vi "Manual Filenames.vi"(8 "Fehler (Eingang)":errorcluster, 9 "Flags Cluster":T4={"PDF Optionen (Eingang)"={"PDF Einzelseiten Komponenten"=FALSE, "PDF Einzelseiten Span"=FALSE, "PDF Deckblatt"=FALSE, "PDF öffnen"=FALSE, "Graphik für Messwerte"=FALSE}, "File Name LIN in"="", "Pfad LIN in"=path "", "active SPAN Idx out"=0, "Comp Idx out"=0, "1. Komponente"=TRUE, "Filename Overrride"=TRUE}, 10 "Zeitstempel":timestamp, 11 "SpanInletClusterArray in":T9[](array[typedef]) {"zusätzliche Zeitdauer Erster Punkt" min=30 step=1 format="%#_5g"; "Zeitdauer Stufen" format="%#_5g"; "Max Fehler" format="%#_5g"; "Anzahl Stufen" format="%#_5g"; "Komponenten"."Komponente 5"."Komponente:" items=["NO (350,3000) LP 191C", "NO2 (150) LP 191C (1of2)", "NO2 (2000) LP 191C (2of2)", "N2O (300) LP 191C (1of2)", "NH3 (300) LP 191C (1of2)", "NH3 (900,3000) LP 191C (2of2)", "HNCO (400) 191C", "H2O% (30) LP 191C", "Formaldehyde (70,500) LP 191C", "CO2 low% (4) LP 191C (2of2)", "CO2% (20) LP 191C (1of2)", "CO (700) LP 191C (1of3)", "CO% (1) LP 191C (2of3)", "Propylene (1000) LP 191C", "Aromatic HC C7 (500) LP 191C", "Ethylene (1000) LP 191C", "CH4 (250) LP 191C (1of2)", "CH4 (5000) LP 191C (2of2)", "Ethane (1000) LP 191C", "Acetylene (1000) LP 191C", "HNO2 (20) 191C", "MeOH (1000) 191C", "CO% (10) LP 191C (3of3)", "Formic Acid (100) 191C", "SO2 (500) LP 191C", "Acetaldehyde (1000) LP 191C", "COS (100) LP 191C", "1,3 butadiene (100) LP 191C", "Oil as Octane (200) LP 191C", "N2O (1000) LP 191C (2of2)", "Propane (200) LP 191C", "NO2 autorange (2000)", "CO autorange (100000)", "CH4 autorange (5000)", "NH3 autorange (3000)", "Temp. Gascell", "Pressure Gascell", "sBeam@2500"]; "Komponenten"."Komponente 5"."Konzentration IST" format="%#.4f"; "Komponenten"."Komponente 5"."Genauigkeit" format="%#.1f"; "Komponenten"."Komponente 4"."Komponente:" items=["NO (350,3000) LP 191C", "NO2 (150) LP 191C (1of2)", "NO2 (2000) LP 191C (2of2)", "N2O (300) LP 191C (1of2)", "NH3 (300) LP 191C (1of2)", "NH3 (900,3000) LP 191C (2of2)", "HNCO (400) 191C", "H2O% (30) LP 191C", "Formaldehyde (70,500) LP 191C", "CO2 low% (4) LP 191C (2of2)", "CO2% (20) LP 191C (1of2)", "CO (700) LP 191C (1of3)", "CO% (1) LP 191C (2of3)", "Propylene (1000) LP 191C", "Aromatic HC C7 (500) LP 191C", "Ethylene (1000) LP 191C", "CH4 (250) LP 191C (1of2)", "CH4 (5000) LP 191C (2of2)", "Ethane (1000) LP 191C", "Acetylene (1000) LP 191C", "HNO2 (20) 191C", "MeOH (1000) 191C", "CO% (10) LP 191C (3of3)", "Formic Acid (100) 191C", "SO2 (500) LP 191C", "Acetaldehyde (1000) LP 191C", "COS (100) LP 191C", "1,3 butadiene (100) LP 191C", "Oil as Octane (200) LP 191C", "N2O (1000) LP 191C (2of2)", "Propane (200) LP 191C", "NO2 autorange (2000)", "CO autorange (100000)", "CH4 autorange (5000)", "NH3 autorange (3000)", "Temp. Gascell", "Pressure Gascell", "sBeam@2500"]; "Komponenten"."Komponente 4"."Konzentration IST" format="%#.4f"; "Komponenten"."Komponente 4"."Genauigkeit" format="%#.1f"; "Komponenten"."Komponente 3"."Komponente:" items=["NO (350,3000) LP 191C", "NO2 (150) LP 191C (1of2)", "NO2 (2000) LP 191C (2of2)", "N2O (300) LP 191C (1of2)", "NH3 (300) LP 191C (1of2)", "NH3 (900,3000) LP 191C (2of2)", "HNCO (400) 191C", "H2O% (30) LP 191C", "Formaldehyde (70,500) LP 191C", "CO2 low% (4) LP 191C (2of2)", "CO2% (20) LP 191C (1of2)", "CO (700) LP 191C (1of3)", "CO% (1) LP 191C (2of3)", "Propylene (1000) LP 191C", "Aromatic HC C7 (500) LP 191C", "Ethylene (1000) LP 191C", "CH4 (250) LP 191C (1of2)", "CH4 (5000) LP 191C (2of2)", "Ethane (1000) LP 191C", "Acetylene (1000) LP 191C", "HNO2 (20) 191C", "MeOH (1000) 191C", "CO% (10) LP 191C (3of3)", "Formic Acid (100) 191C", "SO2 (500) LP 191C", "Acetaldehyde (1000) LP 191C", "COS (100) LP 191C", "1,3 butadiene (100) LP 191C", "Oil as Octane (200) LP 191C", "N2O (1000) LP 191C (2of2)", "Propane (200) LP 191C", "NO2 autorange (2000)", "CO autorange (100000)", "CH4 autorange (5000)", "NH3 autorange (3000)", "Temp. Gascell", "Pressure Gascell", "sBeam@2500"]; "Komponenten"."Komponente 3"."Konzentration IST" format="%#.4f"; "Komponenten"."Komponente 3"."Genauigkeit" format="%#.1f"; "Komponenten"."Komponente 2"."Komponente:" items=["NO (350,3000) LP 191C", "NO2 (150) LP 191C (1of2)", "NO2 (2000) LP 191C (2of2)", "N2O (300) LP 191C (1of2)", "NH3 (300) LP 191C (1of2)", "NH3 (900,3000) LP 191C (2of2)", "HNCO (400) 191C", "H2O% (30) LP 191C", "Formaldehyde (70,500) LP 191C", "CO2 low% (4) LP 191C (2of2)", "CO2% (20) LP 191C (1of2)", "CO (700) LP 191C (1of3)", "CO% (1) LP 191C (2of3)", "Propylene (1000) LP 191C", "Aromatic HC C7 (500) LP 191C", "Ethylene (1000) LP 191C", "CH4 (250) LP 191C (1of2)", "CH4 (5000) LP 191C (2of2)", "Ethane (1000) LP 191C", "Acetylene (1000) LP 191C", "HNO2 (20) 191C", "MeOH (1000) 191C", "CO% (10) LP 191C (3of3)", "Formic Acid (100) 191C", "SO2 (500) LP 191C", "Acetaldehyde (1000) LP 191C", "COS (100) LP 191C", "1,3 butadiene (100) LP 191C", "Oil as Octane (200) LP 191C", "N2O (1000) LP 191C (2of2)", "Propane (200) LP 191C", "NO2 autorange (2000)", "CO autorange (100000)", "CH4 autorange (5000)", "NH3 autorange (3000)", "Temp. Gascell", "Pressure Gascell", "sBeam@2500"]; "Komponenten"."Komponente 2"."Konzentration IST" format="%#.4f"; "Komponenten"."Komponente 2"."Genauigkeit" format="%#.1f"; "Komponenten"."Komponente 1"."Komponente:" items=["NO (350,3000) LP 191C", "NO2 (150) LP 191C (1of2)", "NO2 (2000) LP 191C (2of2)", "N2O (300) LP 191C (1of2)", "NH3 (300) LP 191C (1of2)", "NH3 (900,3000) LP 191C (2of2)", "HNCO (400) 191C", "H2O% (30) LP 191C", "Formaldehyde (70,500) LP 191C", "CO2 low% (4) LP 191C (2of2)", "CO2% (20) LP 191C (1of2)", "CO (700) LP 191C (1of3)", "CO% (1) LP 191C (2of3)", "Propylene (1000) LP 191C", "Aromatic HC C7 (500) LP 191C", "Ethylene (1000) LP 191C", "CH4 (250) LP 191C (1of2)", "CH4 (5000) LP 191C (2of2)", "Ethane (1000) LP 191C", "Acetylene (1000) LP 191C", "HNO2 (20) 191C", "MeOH (1000) 191C", "CO% (10) LP 191C (3of3)", "Formic Acid (100) 191C", "SO2 (500) LP 191C", "Acetaldehyde (1000) LP 191C", "COS (100) LP 191C", "1,3 butadiene (100) LP 191C", "Oil as Octane (200) LP 191C", "N2O (1000) LP 191C (2of2)", "Propane (200) LP 191C", "NO2 autorange (2000)", "CO autorange (100000)", "CH4 autorange (5000)", "NH3 autorange (3000)", "Temp. Gascell", "Pressure Gascell", "sBeam@2500"]; "Komponenten"."Komponente 1"."Konzentration IST" format="%#.4f"; "Komponenten"."Komponente 1"."Genauigkeit" format="%#.1f"; "Ablaufdatum" format="%<%d.%m.%Y>T"; "Gasflasche" items=["----"=10000, "IAG NH3 3000"=0, "IAG NH3 200"=1, "IAG NH3 2000"=2, "IAG MG"=3, "IAG O2"=4]}) -> (0 "Fehler (Ausgang)":errorcluster, 1 "LogInfo-Cluster":T6 {"Gasflasche" items=["----"=10000, "IAG NH3 3000"=0, "IAG NH3 200"=1, "IAG NH3 2000"=2, "IAG MG"=3, "IAG O2"=4]}, 2 "Pfad LIN Cluster":cluster{"Pfad LIN SPAN":T1, "Pfad LIN":path}, 3 "SpanInletClusterArray out":T9[](array[typedef]) {"zusätzliche Zeitdauer Erster Punkt" min=30 step=1 format="%#_5g"; "Zeitdauer Stufen" format="%#_5g"; "Max Fehler" format="%#_5g"; "Anzahl Stufen" format="%#_5g"; "Komponenten"."Komponente 5"."Komponente:" items=["NO (350,3000) LP 191C", "NO2 (150) LP 191C (1of2)", "NO2 (2000) LP 191C (2of2)", "N2O (300) LP 191C (1of2)", "NH3 (300) LP 191C (1of2)", "NH3 (900,3000) LP 191C (2of2)", "HNCO (400) 191C", "H2O% (30) LP 191C", "Formaldehyde (70,500) LP 191C", "CO2 low% (4) LP 191C (2of2)", "CO2% (20) LP 191C (1of2)", "CO (700) LP 191C (1of3)", "CO% (1) LP 191C (2of3)", "Propylene (1000) LP 191C", "Aromatic HC C7 (500) LP 191C", "Ethylene (1000) LP 191C", "CH4 (250) LP 191C (1of2)", "CH4 (5000) LP 191C (2of2)", "Ethane (1000) LP 191C", "Acetylene (1000) LP 191C", "HNO2 (20) 191C", "MeOH (1000) 191C", "CO% (10) LP 191C (3of3)", "Formic Acid (100) 191C", "SO2 (500) LP 191C", "Acetaldehyde (1000) LP 191C", "COS (100) LP 191C", "1,3 butadiene (100) LP 191C", "Oil as Octane (200) LP 191C", "N2O (1000) LP 191C (2of2)", "Propane (200) LP 191C", "NO2 autorange (2000)", "CO autorange (100000)", "CH4 autorange (5000)", "NH3 autorange (3000)", "Temp. Gascell", "Pressure Gascell", "sBeam@2500"]; "Komponenten"."Komponente 5"."Konzentration IST" format="%#.4f"; "Komponenten"."Komponente 5"."Genauigkeit" format="%#.1f"; "Komponenten"."Komponente 4"."Komponente:" items=["NO (350,3000) LP 191C", "NO2 (150) LP 191C (1of2)", "NO2 (2000) LP 191C (2of2)", "N2O (300) LP 191C (1of2)", "NH3 (300) LP 191C (1of2)", "NH3 (900,3000) LP 191C (2of2)", "HNCO (400) 191C", "H2O% (30) LP 191C", "Formaldehyde (70,500) LP 191C", "CO2 low% (4) LP 191C (2of2)", "CO2% (20) LP 191C (1of2)", "CO (700) LP 191C (1of3)", "CO% (1) LP 191C (2of3)", "Propylene (1000) LP 191C", "Aromatic HC C7 (500) LP 191C", "Ethylene (1000) LP 191C", "CH4 (250) LP 191C (1of2)", "CH4 (5000) LP 191C (2of2)", "Ethane (1000) LP 191C", "Acetylene (1000) LP 191C", "HNO2 (20) 191C", "MeOH (1000) 191C", "CO% (10) LP 191C (3of3)", "Formic Acid (100) 191C", "SO2 (500) LP 191C", "Acetaldehyde (1000) LP 191C", "COS (100) LP 191C", "1,3 butadiene (100) LP 191C", "Oil as Octane (200) LP 191C", "N2O (1000) LP 191C (2of2)", "Propane (200) LP 191C", "NO2 autorange (2000)", "CO autorange (100000)", "CH4 autorange (5000)", "NH3 autorange (3000)", "Temp. Gascell", "Pressure Gascell", "sBeam@2500"]; "Komponenten"."Komponente 4"."Konzentration IST" format="%#.4f"; "Komponenten"."Komponente 4"."Genauigkeit" format="%#.1f"; "Komponenten"."Komponente 3"."Komponente:" items=["NO (350,3000) LP 191C", "NO2 (150) LP 191C (1of2)", "NO2 (2000) LP 191C (2of2)", "N2O (300) LP 191C (1of2)", "NH3 (300) LP 191C (1of2)", "NH3 (900,3000) LP 191C (2of2)", "HNCO (400) 191C", "H2O% (30) LP 191C", "Formaldehyde (70,500) LP 191C", "CO2 low% (4) LP 191C (2of2)", "CO2% (20) LP 191C (1of2)", "CO (700) LP 191C (1of3)", "CO% (1) LP 191C (2of3)", "Propylene (1000) LP 191C", "Aromatic HC C7 (500) LP 191C", "Ethylene (1000) LP 191C", "CH4 (250) LP 191C (1of2)", "CH4 (5000) LP 191C (2of2)", "Ethane (1000) LP 191C", "Acetylene (1000) LP 191C", "HNO2 (20) 191C", "MeOH (1000) 191C", "CO% (10) LP 191C (3of3)", "Formic Acid (100) 191C", "SO2 (500) LP 191C", "Acetaldehyde (1000) LP 191C", "COS (100) LP 191C", "1,3 butadiene (100) LP 191C", "Oil as Octane (200) LP 191C", "N2O (1000) LP 191C (2of2)", "Propane (200) LP 191C", "NO2 autorange (2000)", "CO autorange (100000)", "CH4 autorange (5000)", "NH3 autorange (3000)", "Temp. Gascell", "Pressure Gascell", "sBeam@2500"]; "Komponenten"."Komponente 3"."Konzentration IST" format="%#.4f"; "Komponenten"."Komponente 3"."Genauigkeit" format="%#.1f"; "Komponenten"."Komponente 2"."Komponente:" items=["NO (350,3000) LP 191C", "NO2 (150) LP 191C (1of2)", "NO2 (2000) LP 191C (2of2)", "N2O (300) LP 191C (1of2)", "NH3 (300) LP 191C (1of2)", "NH3 (900,3000) LP 191C (2of2)", "HNCO (400) 191C", "H2O% (30) LP 191C", "Formaldehyde (70,500) LP 191C", "CO2 low% (4) LP 191C (2of2)", "CO2% (20) LP 191C (1of2)", "CO (700) LP 191C (1of3)", "CO% (1) LP 191C (2of3)", "Propylene (1000) LP 191C", "Aromatic HC C7 (500) LP 191C", "Ethylene (1000) LP 191C", "CH4 (250) LP 191C (1of2)", "CH4 (5000) LP 191C (2of2)", "Ethane (1000) LP 191C", "Acetylene (1000) LP 191C", "HNO2 (20) 191C", "MeOH (1000) 191C", "CO% (10) LP 191C (3of3)", "Formic Acid (100) 191C", "SO2 (500) LP 191C", "Acetaldehyde (1000) LP 191C", "COS (100) LP 191C", "1,3 butadiene (100) LP 191C", "Oil as Octane (200) LP 191C", "N2O (1000) LP 191C (2of2)", "Propane (200) LP 191C", "NO2 autorange (2000)", "CO autorange (100000)", "CH4 autorange (5000)", "NH3 autorange (3000)", "Temp. Gascell", "Pressure Gascell", "sBeam@2500"]; "Komponenten"."Komponente 2"."Konzentration IST" format="%#.4f"; "Komponenten"."Komponente 2"."Genauigkeit" format="%#.1f"; "Komponenten"."Komponente 1"."Komponente:" items=["NO (350,3000) LP 191C", "NO2 (150) LP 191C (1of2)", "NO2 (2000) LP 191C (2of2)", "N2O (300) LP 191C (1of2)", "NH3 (300) LP 191C (1of2)", "NH3 (900,3000) LP 191C (2of2)", "HNCO (400) 191C", "H2O% (30) LP 191C", "Formaldehyde (70,500) LP 191C", "CO2 low% (4) LP 191C (2of2)", "CO2% (20) LP 191C (1of2)", "CO (700) LP 191C (1of3)", "CO% (1) LP 191C (2of3)", "Propylene (1000) LP 191C", "Aromatic HC C7 (500) LP 191C", "Ethylene (1000) LP 191C", "CH4 (250) LP 191C (1of2)", "CH4 (5000) LP 191C (2of2)", "Ethane (1000) LP 191C", "Acetylene (1000) LP 191C", "HNO2 (20) 191C", "MeOH (1000) 191C", "CO% (10) LP 191C (3of3)", "Formic Acid (100) 191C", "SO2 (500) LP 191C", "Acetaldehyde (1000) LP 191C", "COS (100) LP 191C", "1,3 butadiene (100) LP 191C", "Oil as Octane (200) LP 191C", "N2O (1000) LP 191C (2of2)", "Propane (200) LP 191C", "NO2 autorange (2000)", "CO autorange (100000)", "CH4 autorange (5000)", "NH3 autorange (3000)", "Temp. Gascell", "Pressure Gascell", "sBeam@2500"]; "Komponenten"."Komponente 1"."Konzentration IST" format="%#.4f"; "Komponenten"."Komponente 1"."Genauigkeit" format="%#.1f"; "Ablaufdatum" format="%<%d.%m.%Y>T"; "Gasflasche" items=["----"=10000, "IAG NH3 3000"=0, "IAG NH3 200"=1, "IAG NH3 2000"=2, "IAG MG"=3, "IAG O2"=4]}, 4 "File Name LIN":T3, 5 "Span_Name":string, 6 "File Name EPA":T3 caption="File Name", 7 "File Names":T5)   [LabVIEW 2020, in "Linearisierung v2.lvlib" / "SpanEinstellungen.lvlib"]
uses:
  SpanEinstellungen.lvlib
  Visualisierungs Elemente/String - Eingabefeld.ctl
  SpanInletCluster.ctl
  Seiten/System Einstellungen V2/Konfig Gasflasche.ctl
  Seiten/System Einstellungen V2/Analysatoren.ctl
  Seiten/System Einstellungen V2/Gasflasche Auswahl.ctl
  Komponentencluster mit Formel.ctl
  Komponentenauswahl mit Formel.ctl
  Einheit.ctl
  Seiten/System Einstellungen V2/Traegergas.ctl
  ErrorLogInfoCluster.ctl
  Visualisierungs Elemente/String - Ausgabefeld.ctl
  PDF Optionen.ctl
  Visualisierungs Elemente/Pfad-Eingabefeld.ctl
  <vilib>/regexp/Match Regular Expression.xnode
  Allgemein/allgemeine Sub-VIs.lvlib
  Seiten/System Einstellungen V2/System Einstellungen V2.lvlib
panel:
  out "Deckblatt LIN":string
  out "Deckblatt EPA":string
  # "sec"
  # "%"
  # "sec"
  # "Komponente"
  # "Formel"
  # "Konzentration"
  # "Einheit"
  # "Genauigkeit [%]"
  # "sec"
  # "%"
  # "sec"
  # "Komponente"
  # "Formel"
  # "Konzentration"
  # "Einheit"
  # "Genauigkeit [%]"
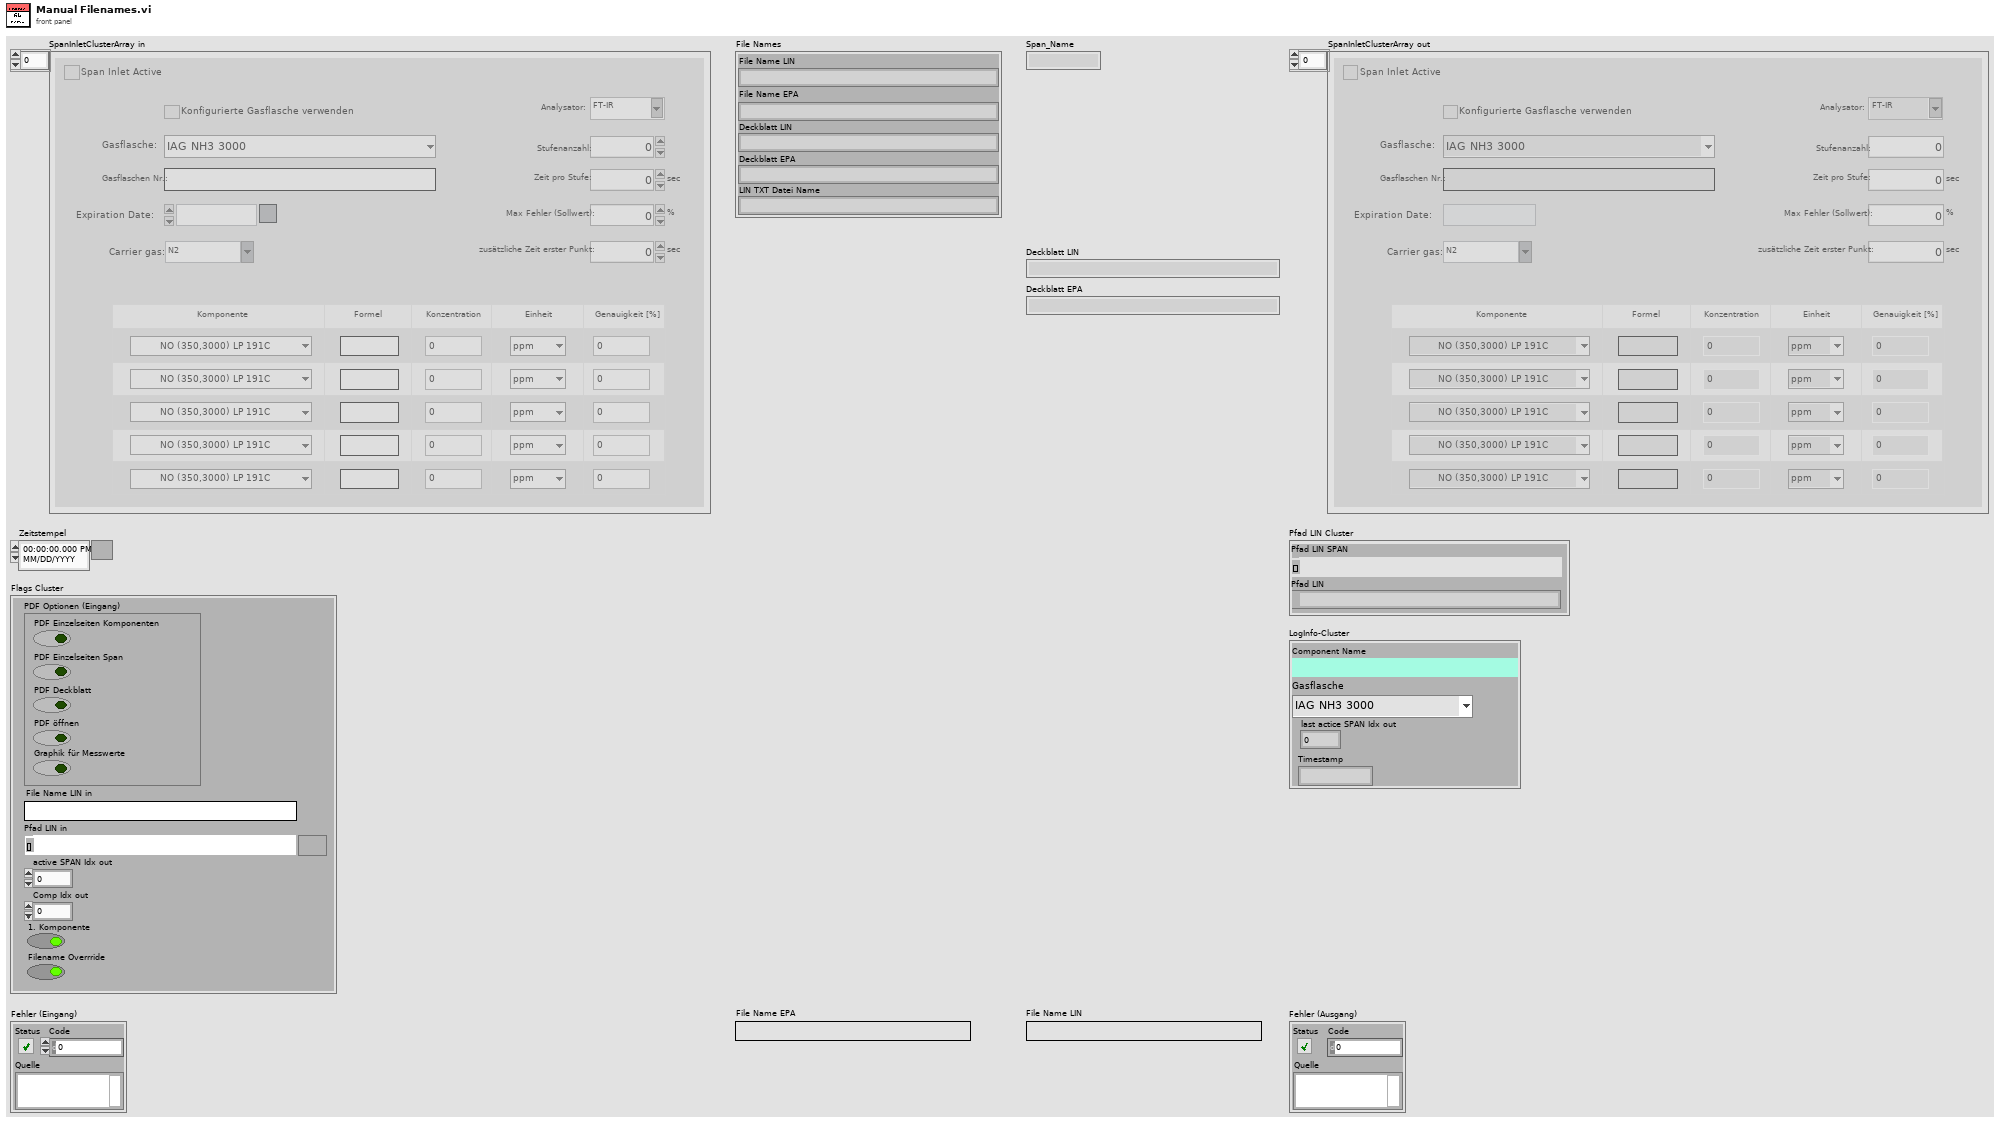
[diagram p1: front panel]
types:
  T1 = typedef "Pfad-Eingabefeld.ctl" = path
  T2 = typedef "Linearisierung v2.lvlib/SpanEinstellungen.lvlib/PDF Optionen.ctl" = cluster{"PDF Einzelseiten Komponenten":bool, "PDF Einzelseiten Span":bool, "PDF Deckblatt":bool, "PDF öffnen":bool, "Graphik für Messwerte":bool}
  T3 = typedef "String - Eingabefeld.ctl" = string
  T4 = cluster{"PDF Optionen (Eingang)":T2, "File Name LIN in":T3, "Pfad LIN in":T1, "active SPAN Idx out":i32, "Comp Idx out":i32, "1. Komponente":bool, "Filename Overrride":bool}
  T5 = cluster{"File Name LIN":string, "File Name EPA":string, "Deckblatt LIN":string, "Deckblatt EPA":string, "LIN TXT Datei Name":string}
  T6 = typedef "Linearisierung v2.lvlib/SpanEinstellungen.lvlib/ErrorLogInfoCluster.ctl" = cluster{"Component Name":T7, "Gasflasche":T8, "last actice SPAN Idx out":i32, "Timestamp":string}
  T7 = typedef "String - Ausgabefeld.ctl" = string
  T8 = typedef "System Einstellungen V2.lvlib/Gasflasche Auswahl.ctl" = u16
  T9 = typedef "Linearisierung v2.lvlib/SpanEinstellungen.lvlib/SpanInletCluster.ctl" = cluster{"Span Inlet Active":T10, "Analysator":T11, "Konfig Gasflasche":T10, "Gasflasche":T8, "Gasflaschen Nr.:":string, "Ablaufdatum":timestamp, "Komponenten":T12, "Zeitdauer Stufen":sgl, "Max Fehler":sgl, "Anzahl Stufen":sgl, "Trägergas":T15, "zusätzliche Zeitdauer Erster Punkt":sgl}
  T10 = typedef "System Einstellungen V2.lvlib/Konfig Gasflasche.ctl" = bool
  T11 = typedef "System Einstellungen V2.lvlib/Analysatoren.ctl" = string
  T12 = typedef "Linearisierung v2.lvlib/SpanEinstellungen.lvlib/Komponentencluster mit Formel.ctl" = cluster{"Komponente 1":T13, "Komponente 2":T13, "Komponente 3":T13, "Komponente 4":T13, "Komponente 5":T13}
  T13 = typedef "Linearisierung v2.lvlib/SpanEinstellungen.lvlib/Komponentenauswahl mit Formel.ctl" = cluster{"Komponente:":u16, "Summenformel":T3, "Konzentration IST":dbl, "Einheit":T14, "Genauigkeit":dbl}
  T14 = typedef "Linearisierung v2.lvlib/SpanEinstellungen.lvlib/Einheit.ctl" = enum16{"ppm", "%"}
  T15 = typedef "System Einstellungen V2.lvlib/Traegergas.ctl" = string
  T16 = cluster{"Component Name":T7, "Compnent Nr":u16, "Formelname(n)":string}
  T17 = cluster{"File Name LIN":string, "File Name EPA":string, "MG":bool}
  T18 = cluster{"Component Name":T7, "Gasflasche":T8, "active SPAN Idx out":i32, "date/time string":string}
  T19 = cluster{"File Name LIN in":T3, "File Name LIN in":T3, string, string, "File Name LIN":string}
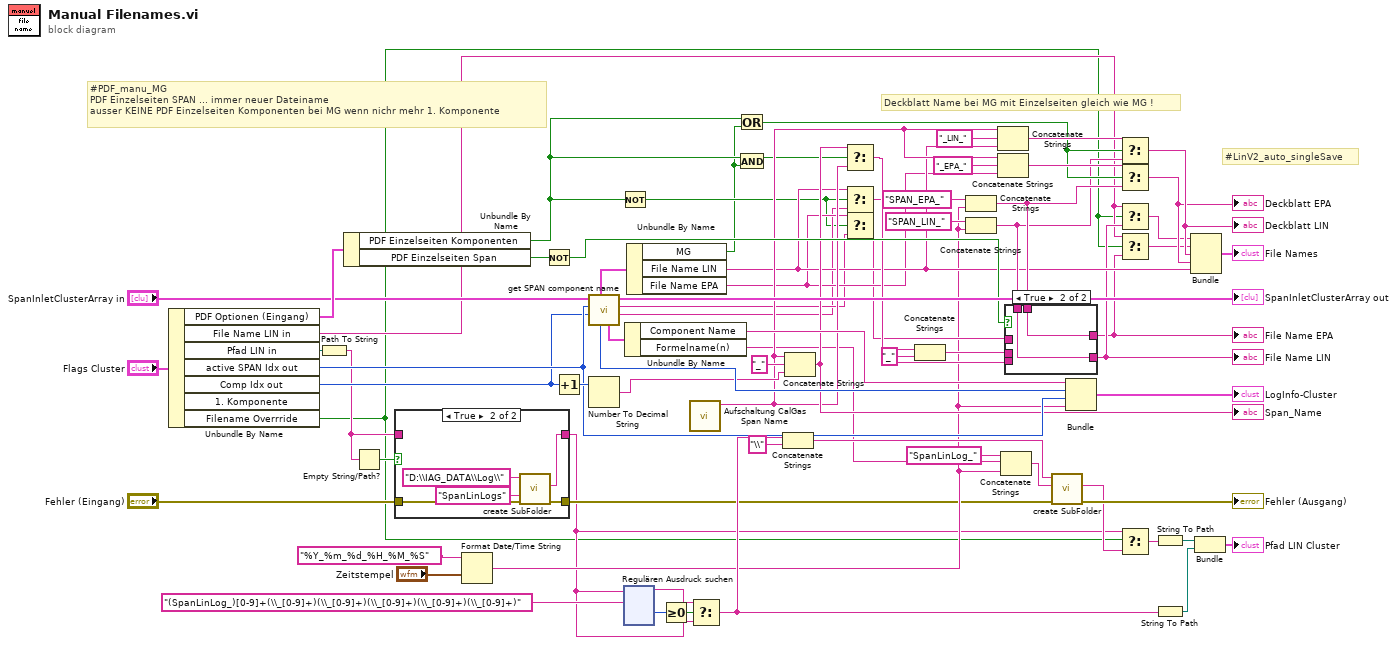
[diagram p0: block diagram]
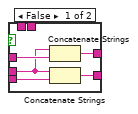
[diagram p3: hidden frame]
diagram:
  # "#LinV2_auto_singleSave"
  # "Deckblatt Name bei MG mit Einzelseiten gleich wie MG !"
  # "#PDF_manu_MG\nPDF Einzelseiten SPAN ... immer neuer Dateiname\nausser KEINE PDF Einzelseiten Komponenten bei MG wenn nichr mehr 1. Komponente"
  n1 = Unbundle By Name("Flags Cluster") -> ("PDF Optionen (Eingang)"=w60:T2, "File Name LIN in"=w5:T3, "Pfad LIN in"=w55:T1, "active SPAN Idx out"=w57:i32, "Comp Idx out"=w56:i32, "Filename Overrride"=w1:bool)  [unwired: 1 out]
  n2 = Path To String(path=w55) -> (string=w14:string)
  n3 = Unbundle By Name(w60) -> ("PDF Einzelseiten Komponenten"=w12:bool, "PDF Einzelseiten Span"=w53:bool)
  n4 = Empty String/Path?(string/path=w14) -> (empty?=w13:bool)
  n5 = case shown="True" w13 {
    tunnel: [w74 w80] -> w15
    tunnel: "Fehler (Eingang)" -> [w74 w79]
    tunnel: w14 -> [w75 _]
    tunnel: [w75 w76] -> w3
    frame False {
    }
    frame True {
      n6 = call "create SubFolder.vi"("Fehler (Eingang)"=w79, "Ordner"="SpanLinLogs", "Pfad"="D:\\IAG_DATA\\Log\\") -> ("Fehler (Ausgang)"=w80:errorcluster, "SubOrdner"=w76:string)  [unwired: 6 in, 1 out]
    }
  }
  n7 = Format Date/Time String(time format string (%c)="%Y_%m_%d_%H_%M_%S" ("Zeitformatierungs-String (%c)"), seconds (now)="Zeitstempel") -> (date/time string=w18:string)  [unwired: 1 in]
  n8 = Not(x=w53) -> (.not. x?=w50:bool)
  n9 = Increment(x=w56) -> (x+1=w65:i32)
  n10 = call "get SPAN component name.vi"("Comp Idx"=w56, "SPAN Idx"=w57, "SpanInletClusterArray in"="SpanInletClusterArray in") -> ("Protokoll Name LIN"=w30:string, "Protokoll Name EPA"=w31:string, "Komponente Nr Name -Cluster"=w69:T16, "Gasflasche"=w68:T8, "LIN/EPA TXT Datei Name"=w54:T17)  [unwired: 1 in, 3 out]
  n11 = Number To Decimal String(number=w65) -> (decimal integer string=w47:string)  [unwired: 1 in]
  n12 = Not(x=w12) -> (.not. x?=w27:bool)
  n13 = xnode "Regulären Ausdruck suchen"("Eingangs-String"=w3, "Regulärer Ausdruck"="(SpanLinLog_)[0-9]+(\\_[0-9]+)(\\_[0-9]+)(\\_[0-9]+)(\\_[0-9]+)(\\_[0-9]+)" ("Ordner")) -> ("Vor Übereinstimmung"=w20:string, "Offset nach Übereinstimmung"=w23:i32)  [unwired: 4 in, 3 out]
  n14 = Unbundle By Name(w69) -> ("Component Name"=w52:T7, "Formelname(n)"=w17:string)
  n15 = Unbundle By Name(w54) -> ("MG"=w10:bool, "File Name LIN"=w34:string, "File Name EPA"=w32:string)
  n16 = Greater Or Equal To 0?(x=w23) -> (x >= 0?=w21:bool)
  n17 = call "Aufschaltung CalGas Span Name.vi"() -> ("Span Name"=w35:T3)  [unwired: 11 in]
  n18 = Select(t=w20, s=w21, f=w3) -> (s? t:f=w19:string)
  n19 = Or(x=w12, y=w10) -> (x .or. y?=w41:bool)
  n20 = And(x=w12, y=w10) -> (x .and. y?=w11:bool)
  n21 = Concatenate Strings(w19, "\\" ("String")) -> (w59:string)
  n22 = Concatenate Strings(w35, "_" ("String"), w47) -> (w46:string)
  "Span_Name" <- w46
  n23 = Select(t=w46, s=w11, f=w35) -> (s? t:f=w36:T3)
  n24 = Select(t=w34, s=w27, f=w30) -> (s? t:f=w28:string)
  n25 = Select(t=w32, s=w27, f=w31) -> (s? t:f=w29:string)
  n26 = Concatenate Strings(w36, "_" ("String")) -> (w64:string)
  n27 = Concatenate Strings("SPAN_EPA_", w18) -> (w40:string)
  n28 = Concatenate Strings("SPAN_LIN_", w18) -> (w39:string)
  n29 = Concatenate Strings(w35, "_LIN_" ("String"), w34) -> (w44:string)
  n30 = Concatenate Strings(w35, "_EPA_" ("String"), w32) -> (w43:string)
  n31 = Concatenate Strings("SpanLinLog_" ("Ordner"), w17, w18) -> (w58:string)
  n32 = case shown="True" w50 {
    tunnel: w28 -> [w85 _]
    tunnel: [w84 w86] -> w9
    tunnel: w29 -> [w83 _]
    tunnel: w64 -> [w82 _]
    tunnel: [w81 w87] -> w7
    tunnel: w40 -> [_ w87]
    tunnel: w39 -> [_ w86]
    frame False {
      n33 = Concatenate Strings(w82, w83) -> (w81:string)
      n34 = Concatenate Strings(w82, w85) -> (w84:string)
    }
    frame True {
    }
  }
  "File Name LIN" <- w9
  "File Name EPA" <- w7
  n35 = call "create SubFolder.vi"("Fehler (Eingang)"=w15, "Ordner"=w58, "Pfad"=w59) -> ("Fehler (Ausgang)"=→"Fehler (Ausgang)":errorcluster, "SubOrdner"=w4:string)  [unwired: 6 in, 1 out]
  n36 = Bundle("Component Name"=w52, "Gasflasche"=w68, "active SPAN Idx out"=w57, "date/time string"=w18) -> (→"LogInfo-Cluster":T18)  [unwired: 1 in]
  n37 = Select(t=w44, s=w41, f=w39) -> (s? t:f=w38:string)
  "Deckblatt LIN" <- w38
  n38 = Select(t=w43, s=w41, f=w40) -> (s? t:f=w37:string)
  "Deckblatt EPA" <- w37
  n39 = Select(t=w5, s=w1, f=w9) -> (s? t:f=w8:T3)
  n40 = Select(t=w5, s=w1, f=w7) -> (s? t:f=w6:T3)
  n41 = Select(t=w3, s=w1, f=w4) -> (s? t:f=w2:string)
  n42 = String To Path(string=w2) -> (path=w26:path)
  n43 = String To Path(string=w19) -> (path=w25:path)
  n44 = Bundle("File Name LIN in"=w8, "File Name LIN in"=w6, w38, w37, "File Name LIN"=w34) -> (→"File Names":T19)  [unwired: 1 in]
  n45 = Bundle(w26, w25) -> (→"Pfad LIN Cluster":cluster{path, path})  [unwired: 1 in]
  "SpanInletClusterArray out" <- "SpanInletClusterArray in"
